vi "niP2P Handle Events.vi"   [LabVIEW 2010]
doc: "Creates an Event structure configured with an Event Dynamic Registration terminal so you can create event cases to handle peer-to-peer streaming events."
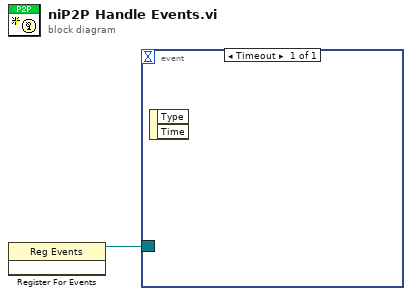
[diagram p0: block diagram]
diagram:
  n1 = register-events() -> (reference out=w1:refnum<event-registration>)  [unwired: 3 in, 1 out]
  n2 = event shown="[0] Timeout" {
    selector: w1 -> [_]
    dyn-events: _ -> [_]
    timeout: _ -> [_]
    event Timeout {
      n3 = event-data() -> ()  [unwired: 1 in, 2 out]
    }
  }
